vi "Savitzky Golay Filter PtByPt.vi"(2 "initialize":bool, 3 "order polynomial":i32=3, 4 "side points":i32=6, 5 "x":dbl format="%0.2f") -> (0 "error":i32, 1 "Filtered x":dbl format="%0.2f")   [LabVIEW 2020, in "NI_PtbyPt.lvlib"]
doc: "Performs fitting based on a polynomial of a given order and then smooths the curve instead of returning raw data."
uses:
  NI_PtbyPt.lvlib
  Real A x B.vi
  Real Inverse Matrix.vi
  NI_AALBase.lvlib
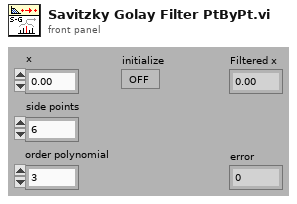
[diagram p1: front panel]
types:
  T1 = typedef "NI_Matrix.lvlib/RealMatrix.ctl" = dbl[][]
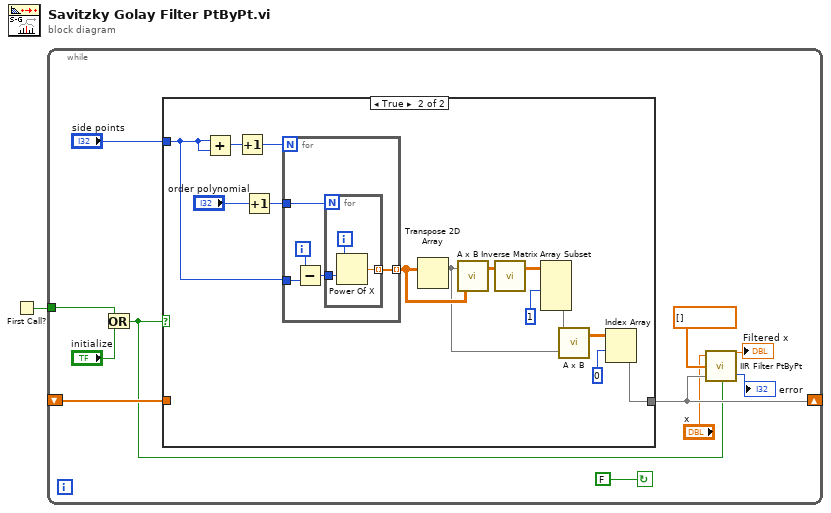
[diagram p0: block diagram]
diagram:
  n1 = First Call?() -> (First Call?: T/F=w1:bool)
  n2 = while {
    tunnel: w1 -> [w5]
    shift-left: _ -> [w12]
    shift-right: [w10] -> _
    stop <- FALSE continue-if-true
    n3 = Or(x=w5, y="initialize") -> (x .or. y?=w3:bool)
    n4 = case shown="True" w3 {
      tunnel: [w13 w17] -> w10
      tunnel: w12 -> [w13 _]
      tunnel: "side points" -> [_ w14]
      frame False {
      }
      frame True {
        n5 = Add(x=w14, y=w14) -> (x+y=w16:i32)
        n6 = Increment(x=w16) -> (x+1=w15:i32)
        n7 = Increment(x="order polynomial") -> (x+1=w26:i32)
        n8 = for {
          N: w15 -> [_]
          tunnel: w14 -> [w32]
          tunnel: w26 -> [w30]
          tunnel: [w28] -> w21 mode=indexing
          i -> [w31]
          n9 = Subtract(x=w31, y=w32) -> (x-y=w29:i32)
          n10 = for {
            N: w30 -> [_]
            tunnel: w29 -> [w35]
            tunnel: [w33] -> w28 mode=indexing
            i -> [w34]
            n11 = Power Of X(1:w35, 2:w34) -> (0:w33:dbl)
          }
        }
        n12 = Transpose 2D Array(2D array=w21) -> (transposed array=w20:dbl[][])
        n13 = call-poly "A x B.vi"("B"=w21, "A"=w20) -> ("A x B"=w25:T1)  [unwired: 1 out]
        n14 = call-poly "Inverse Matrix.vi"("Input Matrix"=w25) -> ("Inverse Matrix"=w24:T1)  [unwired: 1 in, 1 out]
        n15 = Array Subset(array=w24, length (row)=1 ("Array Length")) -> (w22:T1)  [unwired: 3 in]
        n16 = call-poly "A x B.vi"("B"=w20, "A"=w22) -> ("A x B"=w19:T1)  [unwired: 1 out]
        n17 = Index Array(array=w19, index (row)=0 ("Index")) -> (element=w17:dbl[])  [unwired: 1 in]
      }
    }
    n18 = call "IIR Filter PtByPt.vi"("initialize"=w3, "Forward Coefficients"=w10, "Reverse Coefficients"=dbl[] [], "x"="x") -> ("error"=→"error":i32, "Filtered x"=→"Filtered x":dbl)
  }
